vi "Configure Set Current.vi"(8 "error in (no error)":errorcluster, 9 "Current Set (0.0 A)":dbl format="%.2g", 10 "Ch Selector":T1, 11 "VISA resource name":refnum<visa-resource-name>) -> (0 "error out":errorcluster, 3 "VISA resource name out":refnum<visa-resource-name>)   [LabVIEW 2020, in "ScientiFic DC Power Supply.lvlib"]
doc: "Configures Set current of the power supply. Specify the set current limit for Your Application"
uses:
  <instrlib>/ScientiFic DC Power Supply/ScientiFic DC Power Supply.lvlib
  <instrlib>/ScientiFic DC Power Supply/Public/Ch Selector.ctl
panel:
  out "concatenated string":string
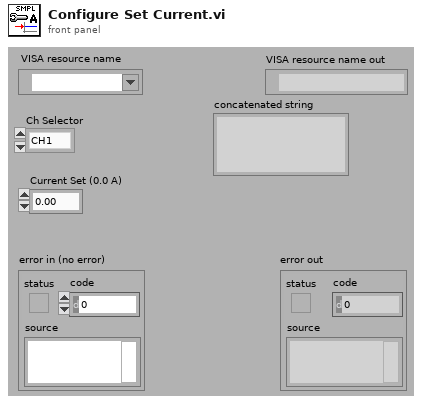
[diagram p1: front panel]
types:
  T1 = typedef "ScientiFic DC Power Supply.lvlib/Ch Selector.ctl" = enum16{"CH1", "CH2", "CH3", "CH4"}
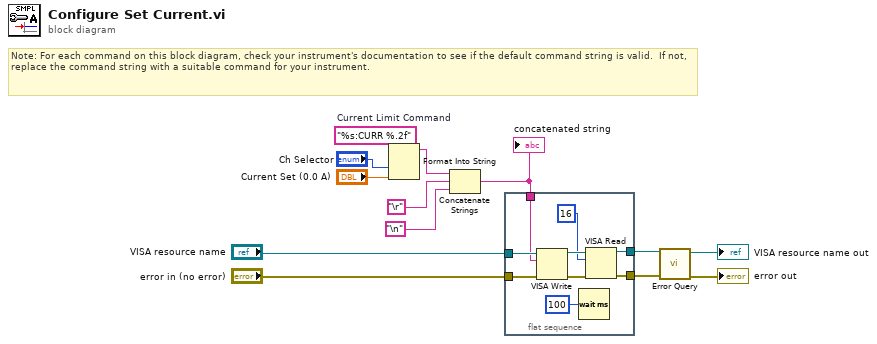
[diagram p0: block diagram]
diagram:
  w8 = "%s:CURR %.2f"  # Current Limit Command
  # "Note: For each command on this block diagram, check your instrument's documentation to see if the default command string is valid.  If not, replace the command string with a suitable command for your instrument."
  n1 = Format Into String(format string=w8, "Ch Selector", "Current Set (0.0 A)") -> (resulting string=w5:string)  [unwired: 2 in, 1 out]
  n2 = Concatenate Strings(w5, "\r", "\n") -> (w4:string)
  "concatenated string" <- w4
  n3 = flat-sequence {
    tunnel: "VISA resource name" -> [w22]
    tunnel: "error in (no error)" -> [w21]
    tunnel: w4 -> [w20]
    tunnel: [w17] -> w3
    tunnel: [w16] -> w2
    frame #0 {
      n4 = VISA Write(VISA resource name=w22, write buffer=w20, error in (no error)=w21) -> (VISA resource name out=w18:refnum<visa-resource-name>, error out=w19:errorcluster)  [unwired: 1 out]
      n5 = Wait (ms)(milliseconds to wait=u32 100) -> ()  [unwired: 1 out]
      n6 = VISA Read(VISA resource name=w18, byte count=u32 16, error in (no error)=w19) -> (VISA resource name out=w17:refnum<visa-resource-name>, error out=w16:errorcluster)  [unwired: 2 out]
    }
  }
  n7 = call <instrlib>:"Error Query.vi"("error in (no error)"=w2, "VISA resource name"=w3) -> ("error out"=→"error out":errorcluster, "VISA resource name out"=→"VISA resource name out":refnum<visa-resource-name>)  [unwired: 8 in]
